vi "Initialize with copy transmission.vi"(8 "error in (no error)":errorcluster, 9 "unit ID":u8=1, 10 "MB copy":refnum<class "WebSocket Client CR.lvclass">, 11 "MB in":refnum<class "WebSocket Client CR.lvclass">) -> (0 "error out":errorcluster, 3 "MB out":refnum<class "WebSocket Client CR.lvclass">)   [LabVIEW 2021, in "WebSockets.lvlib" / "WebSocket Client CR.lvclass"]
uses:
  WebSocket Client CR.lvclass
  WebSocket Client CR.lvclass/WebSocket Client CR.ctl
  Modbus_v121c/Data Model/Device Data Model.lvclass
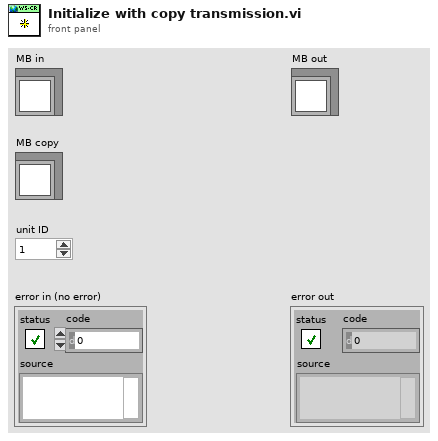
[diagram p1: front panel]
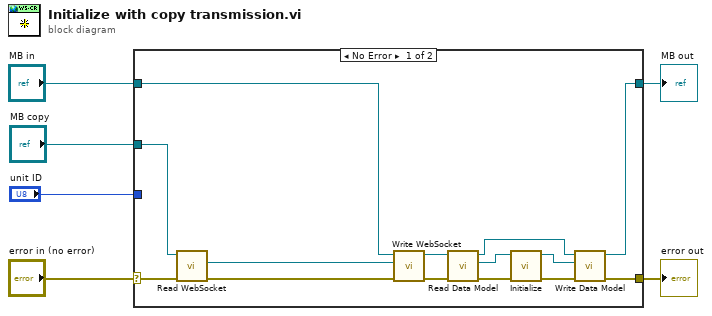
[diagram p0: block diagram]
diagram:
  n1 = case shown="No Error" "error in (no error)" {
    selector: "error in (no error)" -> [w13 w21]
    tunnel: [w14 w21] -> w5
    tunnel: [w15 w22] -> w3
    tunnel: "MB in" -> [w11 w22]
    tunnel: "MB copy" -> [w12 _]
    tunnel: "unit ID" -> [_ _]
    frame No Error {
      n2 = call "Read WebSocket.vi"("error in (no error)"=w13, "Master CR in"=w12) -> ("error out"=w7:errorcluster, "WebSocket"=w8:refnum<class "WebSocket.lvclass">)  [unwired: 7 in, 1 out]
      n3 = call "Write WebSocket.vi"("error in (no error)"=w7, "WebSocket"=w8, "Master CR in"=w11) -> ("error out"=w9:errorcluster, "Master CR out"=w10:refnum<class "WebSocket Client CR.lvclass">)  [unwired: 7 in]
      n4 = call "Read Data Model.vi"("error in (no error)"=w9, "Master CR in"=w10) -> ("error out"=w19:errorcluster, "Data Model"=w20:refnum<class "Device Data Model.lvclass">, "Master CR out"=w16:refnum<class "WebSocket Client CR.lvclass">)  [unwired: 7 in]
      n5 = call-dynamic "Initialize.vi"("error in"=w19, "device data model in"=w20) -> ("error out"=w18:errorcluster, "device data model out"=w17:refnum<class "Device Data Model.lvclass">)  [unwired: 8 in]
      n6 = call "Write Data Model.vi"("error in (no error)"=w18, "Data Model"=w17, "Master CR in"=w16) -> ("error out"=w14:errorcluster, "Master CR out"=w15:refnum<class "WebSocket Client CR.lvclass">)  [unwired: 7 in]
    }
    frame Error {
    }
  }
  "error out" <- w5
  "MB out" <- w3
